vi "newTestStandSeq.vi"(5 "Engine Ref":refnum<k7>, 9 "Requirements":string[](array[string]), 11 "error in (no error)":errorcluster, 12 "Add Req":bool=TRUE) -> (4 "Engine Reference(out)":refnum<k7>, 6 "Sequence File Ref(out)":refnum<k7>, 15 "error out":errorcluster)   [LabVIEW 2010]
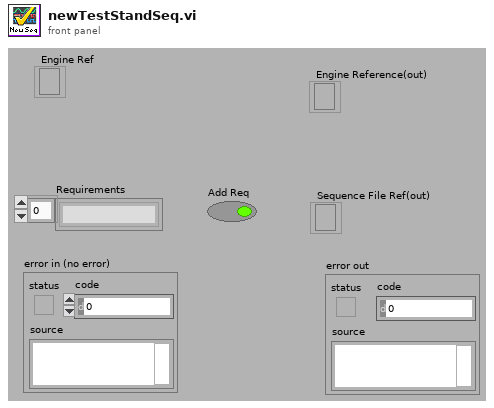
[diagram p1: front panel]
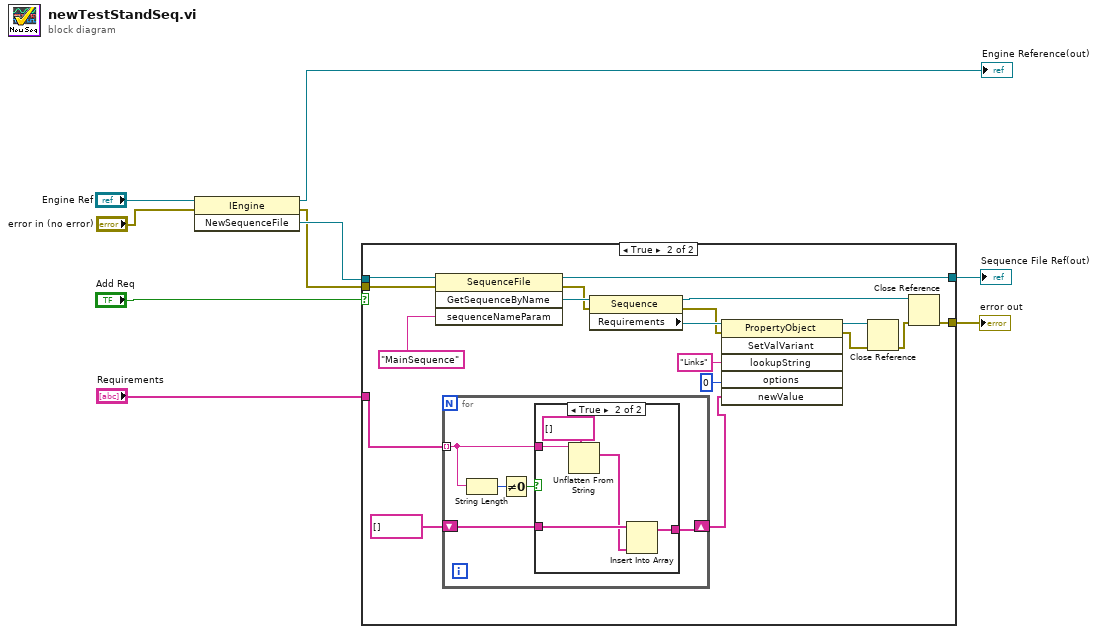
[diagram p0: block diagram]
diagram:
  n1 = invoke class="IEngine" method="NewSequenceFile"(reference="Engine Ref", error in="error in (no error)") -> (reference out=→"Engine Reference(out)":refnum<k7>, error out=w4:errorcluster, "NewSequenceFile"=w5:refnum<k7>)  [unwired: 1 in]
  n2 = case shown="True" "Add Req" {
    tunnel: w5 -> [w11 w29]
    tunnel: w4 -> [w10 w28]
    tunnel: [w11 w27] -> w3
    tunnel: [w10 w17] -> w2
    tunnel: "Requirements" -> [_ w13]
    frame False {
    }
    frame True {
      n3 = invoke class="SequenceFile" method="GetSequenceByName"(reference=w29, error in=w28, "sequenceNameParam"="MainSequence") -> (reference out=w27:refnum<k7>, error out=w24:errorcluster, "GetSequenceByName"=w25:refnum<k7>)  [unwired: 1 in, 1 out]
      n4 = for {
        tunnel: w13 -> [w32] mode=indexing
        shift-right: [w33] -> w12
        shift-left: string[] [] -> [w34]
        n5 = String Length(string=w32) -> (length=w31:i32)
        n6 = Not Equal To 0?(x=w31) -> (x != 0?=w30:bool)
        n7 = case shown="True" w30 {
          tunnel: w34 -> [w35 w39]
          tunnel: [w35 w37] -> w33
          tunnel: w32 -> [_ w36]
          frame False {
          }
          frame True {
            n8 = Unflatten From String(type=string[] [], binary string=w36) -> (value=w38:string[])  [unwired: 3 in, 2 out]
            n9 = Insert Into Array(array=w39, new element=w38) -> (w37:string[])  [unwired: 1 in]
          }
        }
      }
      n10 = property class="Sequence"(reference=w25, error in=w24) -> (reference out=w18:refnum<k7>, error out=w22:errorcluster, "Requirements"=w23:refnum<k7>)
      n11 = invoke class="PropertyObject" method="SetValVariant"(reference=w23, error in=w22, "lookupString"="Links", "options"=0, "newValue"=w12) -> (reference out=w20:refnum<k7>, error out=w21:errorcluster)  [unwired: 1 in, 4 out]
      n12 = Close Reference(reference=w20, error in (no error)=w21) -> (error out=w19:errorcluster)
      n13 = Close Reference(reference=w18, error in (no error)=w19) -> (error out=w17:errorcluster)
    }
  }
  "error out" <- w2
  "Sequence File Ref(out)" <- w3
